vi "TestFile.vi"() -> ()   [LabVIEW 2017]
panel:
  out "Array 8":u8[](array[numeric])
  out "Numeric 2":i32 format="%.0x"
  out "String":string
  out "string":string
  out "Array 7":u8[](array[numeric]) format="%02x"
  out "sumData":u16
  out "y":i32
  out "Array 5":u16[](array[numeric]) format="%04x"
  out "(hi.lo)":u16 format="%.0x"
  out "resulting string 2":string
  out "resulting string":string
  out "x+y 2":i32 format="%.0x"
  out "x .and. y?":u8 format="%.0x"
  out "x+y":u16 format="%.0x"
  in  "Initial Hex String":string="Hello World!"
  out "Normal String - Number to Hexadecimal String Method":string
  out "Array 6":u8[](array[numeric]) format="%02x"
  out "text":string
  out "sum":u16 format="%.0x"
  out "Array 4":u8[](array[numeric])
  out "data string":string
  out "x = y?":bool
  in  "Numeric":u16=263 format="%.0x"
  out "concatenated string":string
  out "ASCII character":string
  in  "ASCII code (U8)":u8=65
  out "Array 3":string[](array[string])
  in  "Array 2":u8[](array[numeric])=[170, 8, 0, 0, 0, 0, 0, 0, 0, 0, 0, 0, 0, 0, 0, 0, 0, 0, 62, 0, 141, 230]
  in  "format string":string
  out "Array":string[](array[string])
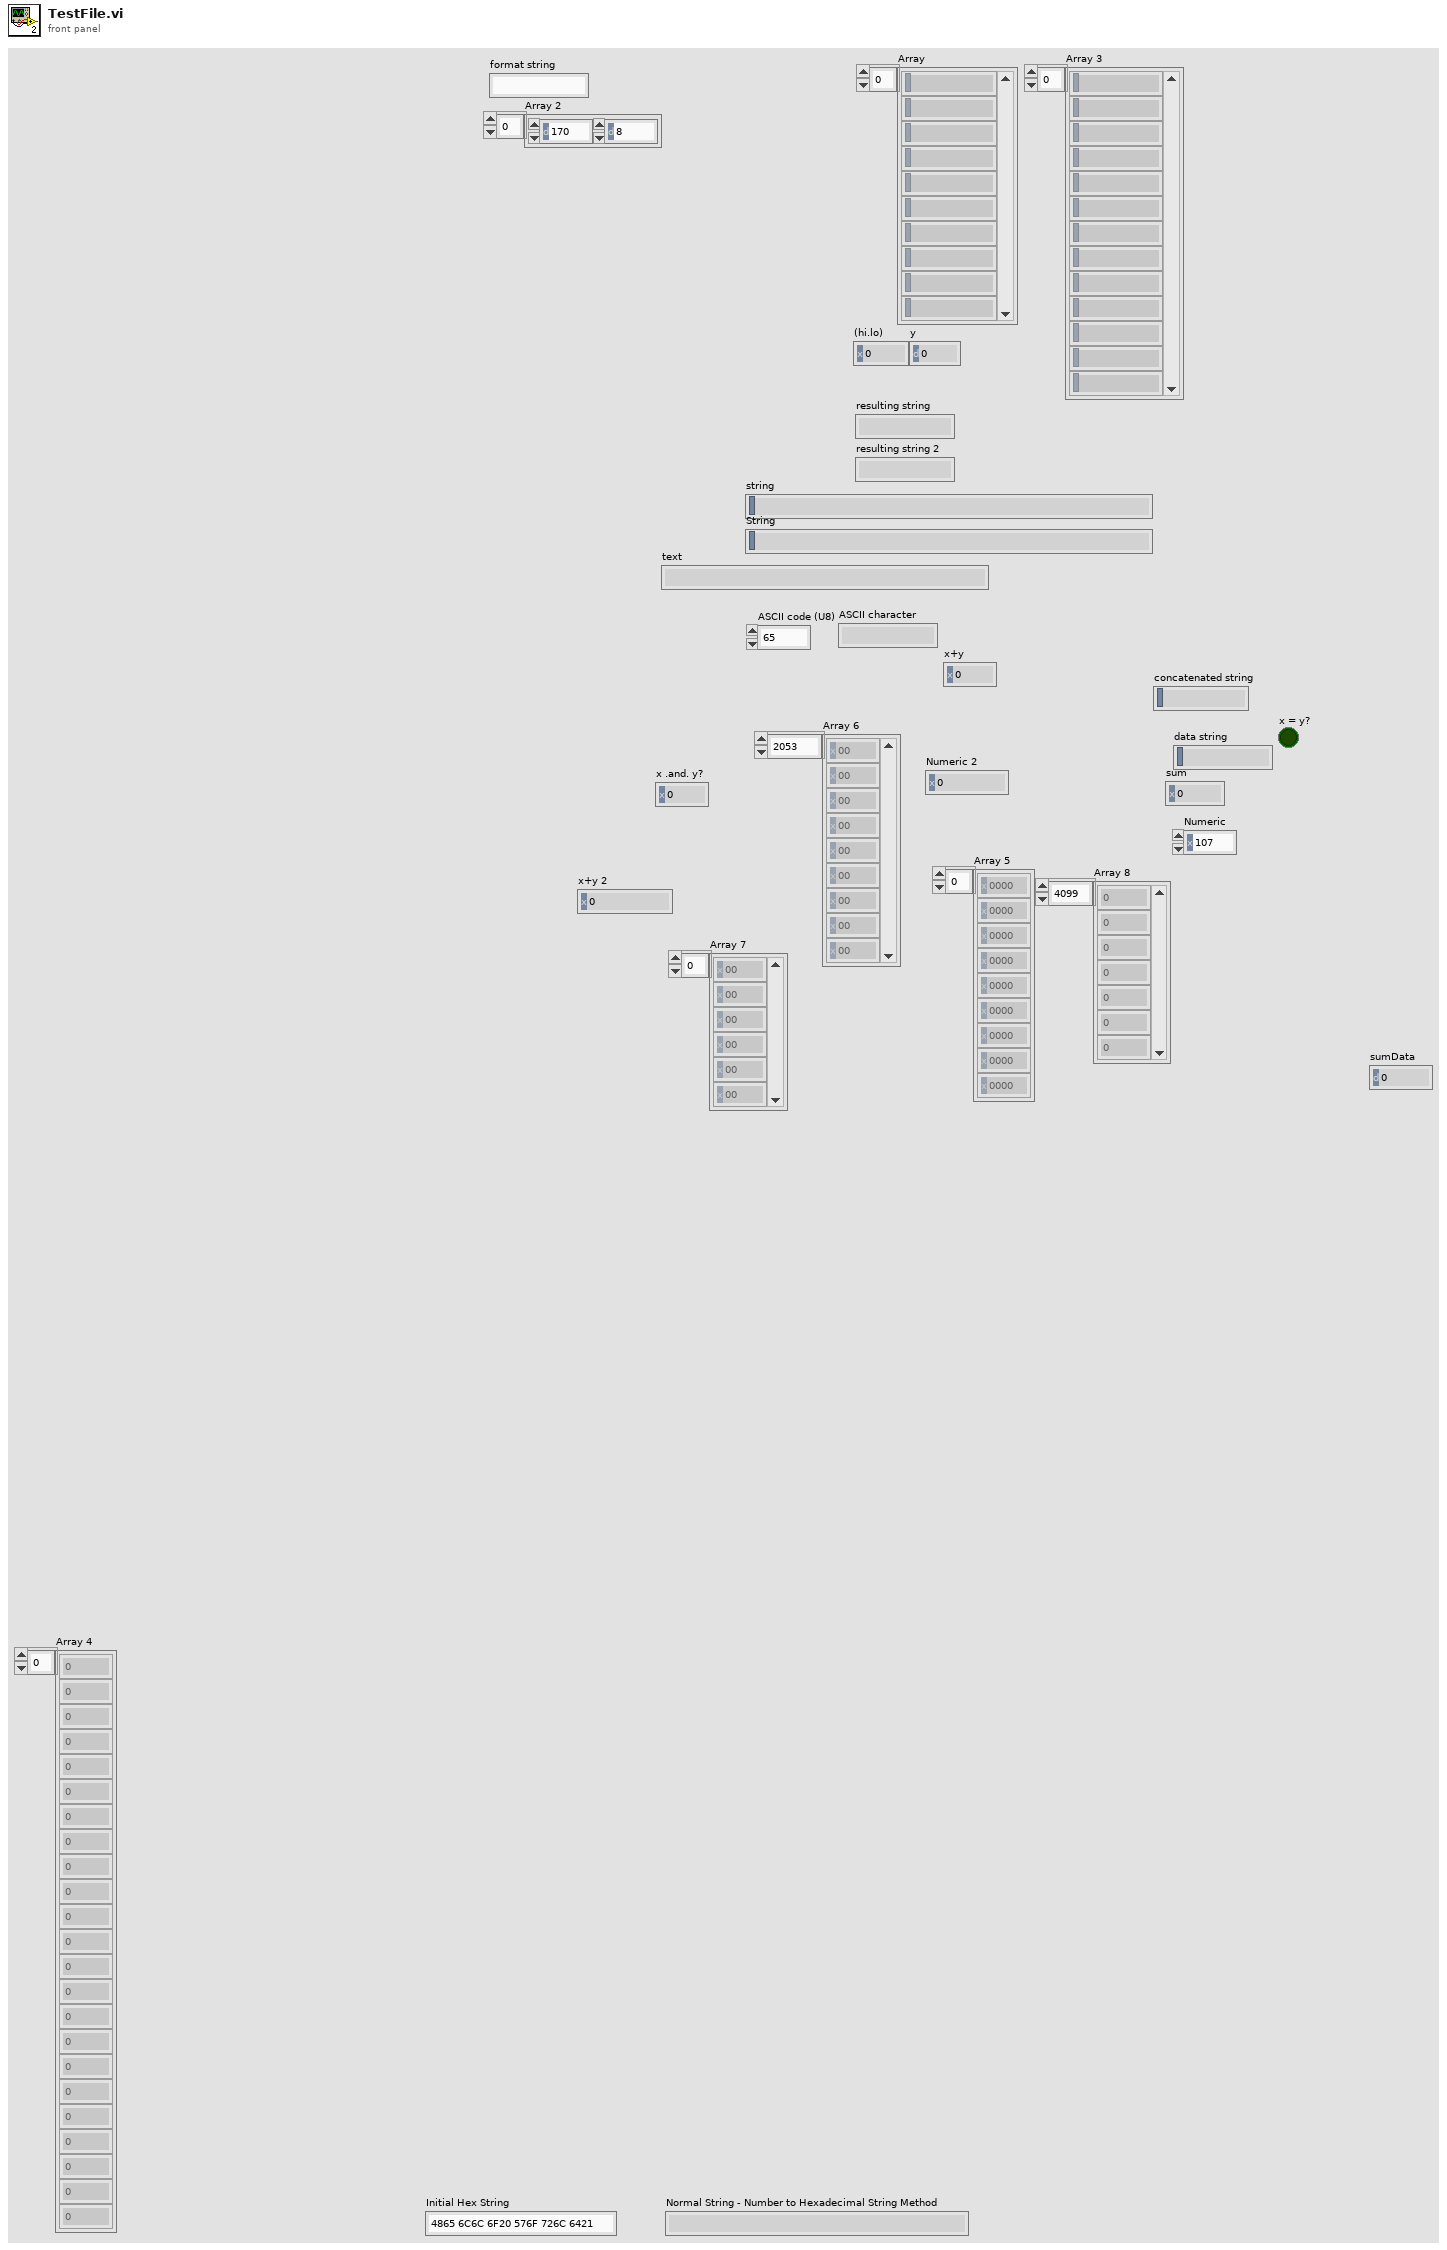
[diagram p1: front panel]
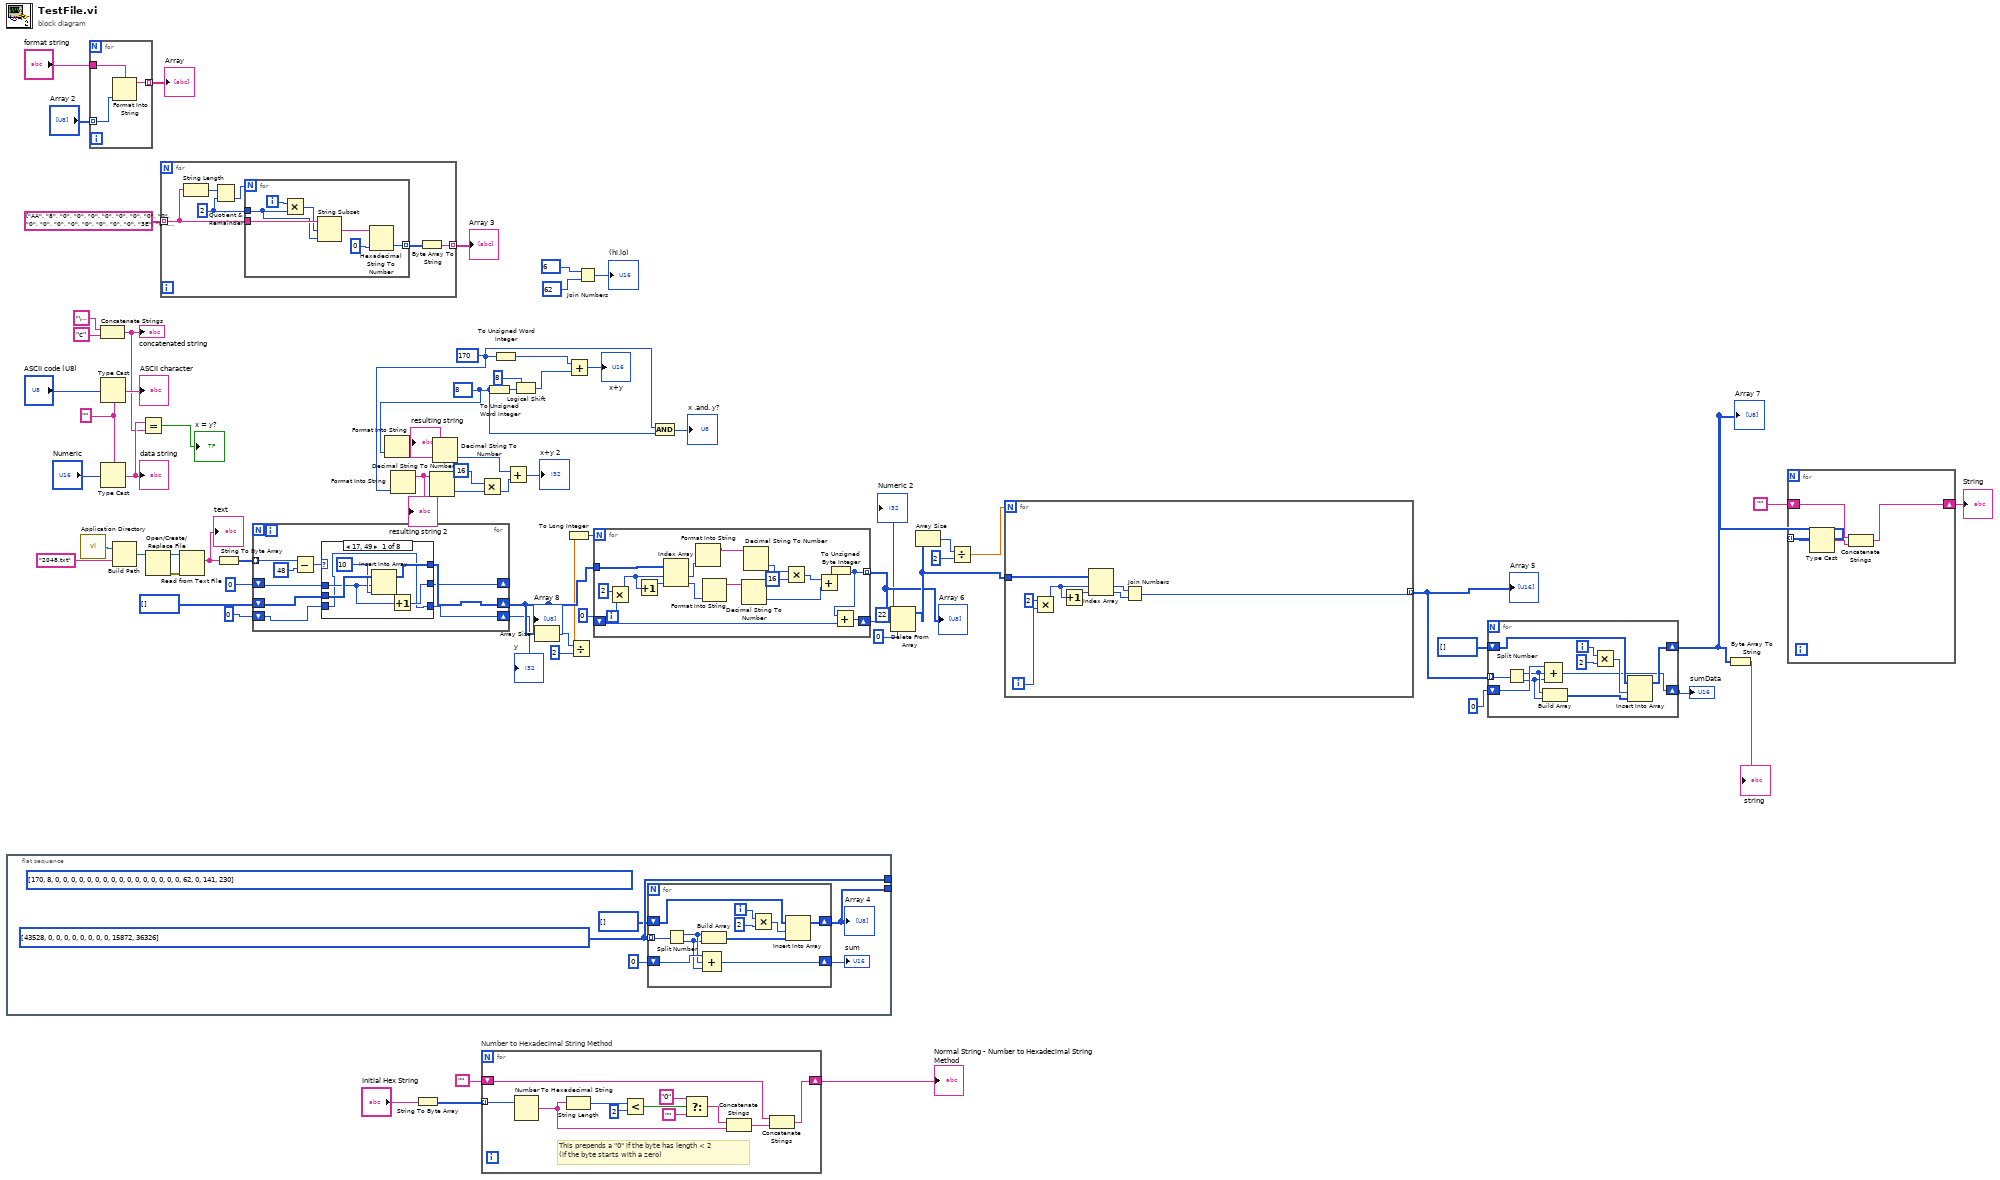
[diagram p0: block diagram]
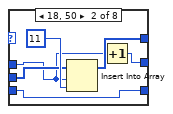
[diagram p2: hidden frame]
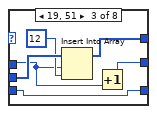
[diagram p3: hidden frame]
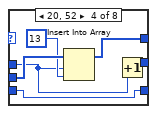
[diagram p4: hidden frame]
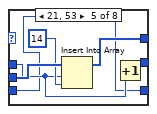
[diagram p5: hidden frame]
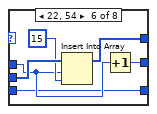
[diagram p6: hidden frame]
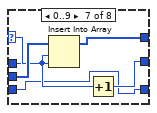
[diagram p7: hidden frame]
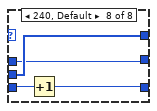
[diagram p8: hidden frame]
diagram:
  w36 = u8 8
  w32 = u8 170
  w58 = "" ("type")
  n1 = flat-sequence {
    tunnel: [w74] -> _
    tunnel: [w70] -> _
    frame #0 {
      w74 = u16[] [43528, 0, 0, 0, 0, 0, 0, 0, 0, 15872, 36326]
      (unwired) u8[] [170, 8, 0, 0, 0, 0, 0, 0, 0, 0, 0, 0, 0, 0, 0, 0, 0, 0, 62, 0, 141, 230]
      n2 = for {
        tunnel: w74 -> [w85] mode=indexing
        shift-right: [w80] -> w70
        shift-left: u8[] [] -> [w79]
        shift-right: [w77] -> w71
        shift-left: u16 0 -> [w78]
        i -> [w84]
        n3 = Split Number(x=w85) -> (hi(x)=w76:u8, lo(x)=w75:u8)
        n4 = Build Array(w76, w75) -> (w82:u8[])
        n5 = Compound Arithmetic op=ADD(w78, w76, w75) -> (w77:u16)
        n6 = Multiply(x=w84, y=2) -> (x*y=w81:i32)
        n7 = Insert Into Array(array=w79, index=w81, new element=w82) -> (w80:u8[])
      }
      "sum" <- w71
      "Array 4" <- w70
    }
  }
  n8 = call <vilib>:"Application Directory.vi"() -> ("Application Directory"=w55:path)
  n9 = for {
    tunnel: "Array 2" -> [w88] mode=indexing
    tunnel: [w87] -> w68 mode=indexing
    tunnel: "format string" -> [w86]
    n10 = Format Into String(format string=w86, w88) -> (resulting string=w87:string)  [unwired: 2 in, 1 out]
  }
  "Array" <- w68
  n11 = Concatenate Strings("\u0002" ("string"), "c" ("string")) -> (w56:string)
  "concatenated string" <- w56
  n12 = Type Cast(type=w58, x="ASCII code (U8)") -> (*(type *) &x=→"ASCII character":string)
  n13 = Type Cast(type=w58, x="Numeric") -> (*(type *) &x=w57:string)
  "data string" <- w57
  n14 = Build Path(base path=w55, name or relative path="2048.txt") -> (appended path=w51:path)
  n15 = Equal?(x=w57, y=w56) -> (x = y?=→"x = y?":bool)
  n16 = Open/Create/Replace File(file path (use dialog)=w51) -> (refnum out=w52:refnum<file>, error out=w53:errorcluster)  [unwired: 5 in, 1 out]
  n17 = for {
    tunnel: [w90] -> w65 mode=indexing
    tunnel: string[] ["AA", "8", "0", "0", "0", "0", "0", "0", "0", "0", "0", "0", "0", "0", "0", "0", "0", "0", "3E", "0", "8D", "E6"] ("Array 2") -> [w89] mode=indexing
    w91 = 2 ("y")
    n18 = String Length(string=w89) -> (length=w93:i32)
    n19 = Quotient & Remainder(x=w93, y=w91) -> (floor(x/y)=w92:i32)  [unwired: 1 out]
    n20 = for {
      N: w92 -> [_]
      tunnel: w89 -> [w99]
      tunnel: [w100] -> w94 mode=indexing
      tunnel: w91 -> [w95]
      i -> [w96]
      n21 = Multiply(x=w96, y=w95) -> (x*y=w97:i32)
      n22 = String Subset(string=w99, offset (0)=w97, length (rest)=w95) -> (substring=w98:string)
      n23 = Hexadecimal String To Number(string=w98, default (0uL)=u8 0) -> (number=w100:u8)  [unwired: 1 in, 1 out]
    }
    n24 = Byte Array To String(unsigned byte array=w94) -> (string=w90:string)
  }
  "Array 3" <- w65
  n25 = Read from Text File(file (use dialog)=w52, error in=w53) -> (text=w49:string)  [unwired: 2 in, 3 out]
  "text" <- w49
  n26 = String To Byte Array(string=w49) -> (unsigned byte array=w50:u8[])
  n27 = for {
    tunnel: w50 -> [w110] mode=indexing
    shift-right: [w106] -> w30
    shift-left: u8[] [] -> [w107]
    shift-right: [w105] -> _
    shift-left: 0 ("y") -> [w104]
    shift-right: [w102] -> w12
    shift-left: 0 ("y") -> [w103]
    n28 = Subtract(x=w110, y=u8 48) -> (x-y=w108:u8)
    n29 = case shown="17, 49" w108 {
      selector: w108 -> [_ _ _ _ _ _ w151 _]
      tunnel: [w114 w120 w127 w132 w138 w144 w150 w156] -> w106
      tunnel: w107 -> [w116 w121 w128 w134 w140 w146 w152 w156]
      tunnel: [w112 w118 w124 w130 w136 w142 w148 w155] -> w105
      tunnel: w104 -> [w113 w119 w125 w131 w137 w143 w149 w155]
      tunnel: w103 -> [w111 w117 w123 w129 w135 w141 w147 w154]
      tunnel: [w111 w117 w123 w129 w135 w141 w147 w153] -> w102
      frame 17, 49 {
        n30 = Insert Into Array(array=w116, index=w113, new element=u8 10) -> (w114:u8[])
        n31 = Increment(x=w113) -> (x+1=w112:i32)
      }
      frame 18, 50 {
        n32 = Insert Into Array(array=w121, index=w119, new element=u8 11) -> (w120:u8[])
        n33 = Increment(x=w119) -> (x+1=w118:i32)
      }
      frame 19, 51 {
        n34 = Insert Into Array(array=w128, index=w125, new element=u8 12) -> (w127:u8[])
        n35 = Increment(x=w125) -> (x+1=w124:i32)
      }
      frame 20, 52 {
        n36 = Insert Into Array(array=w134, index=w131, new element=u8 13) -> (w132:u8[])
        n37 = Increment(x=w131) -> (x+1=w130:i32)
      }
      frame 21, 53 {
        n38 = Insert Into Array(array=w140, index=w137, new element=u8 14) -> (w138:u8[])
        n39 = Increment(x=w137) -> (x+1=w136:i32)
      }
      frame 22, 54 {
        n40 = Insert Into Array(array=w146, index=w143, new element=u8 15) -> (w144:u8[])
        n41 = Increment(x=w143) -> (x+1=w142:i32)
      }
      frame 0..9 {
        n42 = Insert Into Array(array=w152, index=w149, new element=w151) -> (w150:u8[])
        n43 = Increment(x=w149) -> (x+1=w148:i32)
      }
      frame 240, Default {
        n44 = Increment(x=w154) -> (x+1=w153:i32)
      }
    }
  }
  "y" <- w12
  "Array 8" <- w30
  n45 = Format Into String(w36) -> (resulting string=w35:string)  [unwired: 3 in, 1 out]
  "resulting string" <- w35
  n46 = Format Into String(w32) -> (resulting string=w33:string)  [unwired: 3 in, 1 out]
  "resulting string 2" <- w33
  n47 = String To Byte Array(string="Initial Hex String") -> (unsigned byte array=w43:u8[])
  n48 = Decimal String To Number(string=w33) -> (number=w34:i32)  [unwired: 2 in, 1 out]
  n49 = Decimal String To Number(string=w35) -> (number=w18:i32)  [unwired: 2 in, 1 out]
  n50 = Multiply(x=16 ("y"), y=w34) -> (x*y=w20:i32)
  n51 = for "Number to Hexadecimal String Method" {
    shift-right: [w167] -> w45
    shift-left: "" -> [w157]
    tunnel: w43 -> [w158] mode=indexing
    # "This prepends a \"0\" if the byte has length < 2\n(if the byte starts with a zero)"
    n52 = Number To Hexadecimal String(2:w158) -> (0:w160:string)  [unwired: 1 in]
    n53 = String Length(string=w160) -> (length=w166:i32)
    n54 = Less?(x=w166, y=2) -> (x < y?=w164:bool)
    n55 = Select(t="0", s=w164, f="") -> (s? t:f=w161:string)
    n56 = Concatenate Strings(w161, w160) -> (w159:string)
    n57 = Concatenate Strings(w157, w159) -> (w167:string)
  }
  "Normal String - Number to Hexadecimal String Method" <- w45
  n58 = To Unsigned Word Integer(number=w36) -> (unsigned 16bit integer=w42:u16)
  n59 = To Unsigned Word Integer(number=w32) -> (unsigned 16bit integer=w39:u16)
  n60 = Add(x=w18, y=w20) -> (x+y=→"x+y 2":i32)
  n61 = Logical Shift(y=i16 8, x=w42) -> (x << y=w38:u16)
  n62 = Array Size(array=w30) -> (size(s)=w29:i32)
  n63 = Add(x=w39, y=w38) -> (x+y=→"x+y":u16)
  n64 = Divide(x=w29, y=2) -> (x/y=w27:dbl)
  n65 = To Long Integer(number=w27) -> (32bit integer=w26:i32)
  n66 = Join Numbers(hi=u8 6, lo=u8 62) -> ((hi.lo)=→"(hi.lo)":u16)
  n67 = for {
    N: w26 -> [_]
    tunnel: w30 -> [w184]
    tunnel: [w170] -> w3 mode=indexing
    shift-right: [w169] -> w1
    shift-left: 0 -> [w168]
    i -> [w183]
    n68 = Multiply(x=2, y=w183) -> (x*y=w181:i32)
    n69 = Increment(x=w181) -> (x+1=w180:i32)
    n70 = Index Array(array=w184, index #1=w181, index #2=w180) -> (element #1=w173:u8, element #2=w172:u8)
    n71 = Format Into String(w173) -> (resulting string=w174:string)  [unwired: 3 in, 1 out]
    n72 = Format Into String(w172) -> (resulting string=w179:string)  [unwired: 3 in, 1 out]
    n73 = Decimal String To Number(string=w179) -> (number=w178:i32)  [unwired: 2 in, 1 out]
    n74 = Decimal String To Number(string=w174) -> (number=w175:i32)  [unwired: 2 in, 1 out]
    n75 = Multiply(x=w175, y=16) -> (x*y=w177:i32)
    n76 = Add(x=w177, y=w178) -> (x+y=w171:i32)
    n77 = To Unsigned Byte Integer(number=w171) -> (unsigned 8bit integer=w170:u8)
    n78 = Add(x=w170, y=w168) -> (x+y=w169:i32)
  }
  "Array 6" <- w3
  "Numeric 2" <- w1
  n79 = And(x=w32, y=w36) -> (x .and. y?=→"x .and. y?":u8)
  n80 = Delete From Array(array=w3, length=22, index=0) -> (array with subset deleted=w14:u8[])  [unwired: 1 out]
  n81 = Array Size(array=w14) -> (size(s)=w22:i32)
  n82 = Divide(x=w22, y=2) -> (x/y=w21:dbl)
  n83 = for {
    N: w21 -> [_]
    tunnel: w14 -> [w189]
    tunnel: [w185] -> w8 mode=indexing
    i -> [w188]
    n84 = Multiply(x=2, y=w188) -> (x*y=w191:i32)
    n85 = Increment(x=w191) -> (x+1=w192:i32)
    n86 = Index Array(array=w189, index #1=w191, index #2=w192) -> (element #1=w187:u8, element #2=w186:u8)
    n87 = Join Numbers(hi=w187, lo=w186) -> ((hi.lo)=w185:u16)
  }
  "Array 5" <- w8
  n88 = for {
    tunnel: w8 -> [w203] mode=indexing
    shift-right: [w198] -> w6
    shift-left: u8[] [] -> [w197]
    shift-right: [w195] -> w10
    shift-left: u16 0 -> [w196]
    i -> [w202]
    n89 = Split Number(x=w203) -> (hi(x)=w194:u8, lo(x)=w193:u8)
    n90 = Build Array(w194, w193) -> (w200:u8[])
    n91 = Compound Arithmetic op=ADD(w196, w194, w193) -> (w195:u16)
    n92 = Multiply(x=w202, y=2) -> (x*y=w199:i32)
    n93 = Insert Into Array(array=w197, index=w199, new element=w200) -> (w198:u8[])
  }
  "sumData" <- w10
  "Array 7" <- w6
  n94 = Byte Array To String(unsigned byte array=w6) -> (string=→"string":string)
  n95 = for {
    tunnel: w6 -> [w207] mode=indexing
    shift-right: [w204] -> w4
    shift-left: "" -> [w205]
    n96 = Type Cast(x=w207) -> (*(type *) &x=w206:string)  [unwired: 1 in]
    n97 = Concatenate Strings(w205, w206) -> (w204:string)
  }
  "String" <- w4
